vi "Filter Rendering.vi"() -> ()   [LabVIEW 2023]
doc: "Demonstrates how to use the DFD Render Transfer Function Equation VI, DFD Render Zero-Pole-Gain Equation VI, and DFD Render Difference Equation VI to present the characteristics of a filter in different graphs.\n\nComplete the following steps to use this VI.\n1) Run the VI.\n2) On the <B>Transfer Function Rendering</B> page, modify the <B>Transfer Function Display Format</B> option, and view the resulting transfer function. You also can modify the filter specifications.\n3) Click the <B>Zero-Pole-Gain Rendering</B> tab, modify the <B>Zero-Pole-Gain Equation Display Format</B> option, and view the resulting zero-pole-gain equation.\n4) Click the <B>Difference Equation Rendering</B> tab, modify the <B>Difference Equation Display Format</B> option, and view the resulting difference equation.\n5) Click the <B>STOP</B> button to stop this VI."
uses:
  <vilib>/addons/Digital Filter Design/_Objects.llb/DFD Filter Ripple Specification (Design).ctl
  <vilib>/addons/Digital Filter Design/_Objects.llb/DFD Filter Frequence Specification (Design).ctl
  <vilib>/addons/Digital Filter Design/NI_DigFilterLicensed.lvlib
panel:
  in  "Tab Control":T1(tab)
  out "Transfer Function":picture
  in  "Transfer Functions Display Format":u16(ring) items=["Expanded Form", " Second-Order Sections"]
  out "Zero-Pole-Gain Equation":picture
  in  "Zero-Pole-Gain Equation Display Format":u16(ring) items=["Separated Roots", "Combined Roots"]
  out "Difference Equation":picture
  in  "Difference Equation Display Format":u16(ring) items=["Feedback on left and feedforward on right", "Feedback and feedforward on right", "Feedback and feedforward on right in one line"]
  in  "Design Method":T2(ring)=enum."Elliptic"
  in  "Filter Type":u16(ring) items=["Lowpass", "Highpass", "Bandpass", "Bandstop"]
  in  "Frequency Sepcifications [Hz]":T3={"fpass 1"=250.0, "fstop 1"=400.0, "fpass 2 "=0.0, "fstop 2"=0.0}
  in  "Ripple Specifications":T4={"passband"=0.1, "stopband"=60.0, "dB/linear? (T: dB)"=TRUE}
  in  "Sampling Frequency [Hz]":dbl=1000.0 format="%.2f"
  in  "stop":bool
  out "Error Message":string
  # "Select Help>>Show Context Help and move the cursor over the VI icon for more information."
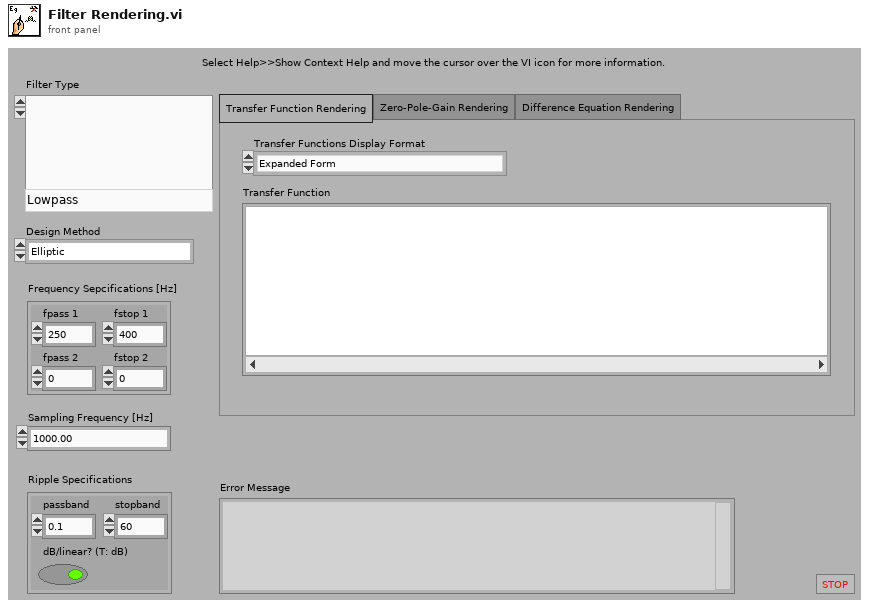
[diagram p1: front panel]
types:
  T1 = enum32{"Transfer Function Rendering", "Zero-Pole-Gain Rendering", "Difference Equation Rendering"}
  T2 = enum16{"Butterworth", "Chebyshev", "Inverse Chebyshev", "Elliptic", "Kaiser Window", "Dolph-Chebyshev Window", "Equi-Ripple FIR"}
  T3 = typedef "NI_DigFilterLicensed.lvlib/DFD Filter Frequence Specification (Design).ctl" = cluster{"fpass 1":dbl, "fstop 1":dbl, "fpass 2 ":dbl, "fstop 2":dbl}
  T4 = typedef "NI_DigFilterLicensed.lvlib/DFD Filter Ripple Specification (Design).ctl" = cluster{"passband":dbl, "stopband":dbl, "dB/linear? (T: dB)":bool}
  T5 = typedef "NI_DigFilterLicensed.lvlib/DFD Filter Obj.ctl" = cluster{"mSRate_Fs":dbl, "mSRate_Version":string, "mSRate_Comments":string, "mSRate_OrgCoef":T6, "mSRate_CurCoef":T6, "mSRate_Quantized?":bool, "mSRate_QCoef":T6, "mSRate_QSettings":T8[], "mSRate_Order":i32, "mSRate_Scaling":cluster{"mSRate_ScaleByPowerOf2?":bool, "mSRate_ScaleType":T10}}
  T6 = typedef "NI_DigFilterLicensed.lvlib/DFD Filter Coef.ctl" = cluster{"type":T7, "gain":dbl, "coef a (k)":dbl[], "coef b (v)":dbl[]}
  T7 = typedef "NI_DigFilterLicensed.lvlib/DFD Filter Structure Type Selector.ctl" = enum16{"Undefined", "FIR Direct Form", "FIR Direct Form Transposed", "FIR Symmetric", "FIR Antisymmetric", "IIR Direct Form I", "IIR Direct Form I Transposed", "IIR Direct Form II", "IIR Direct Form II Transposed", "IIR Cascaded Second Order Sections Form I", "IIR Cascaded Second Order Sections Form I Transposed", "IIR Cascaded Second Order Sections Form II", "IIR Cascaded Second Order Sections Form II Transposed", "Lattice Allpass (basic sections)", "Lattice Allpass (one multiplier sections)", "Lattice Allpass (normalized sections)", "Lattice AR (basic sections)", "Lattice AR (one multiplier sections)", "Lattice AR (normalized sections)", "Lattice MA (minimum phase)", "Lattice MA (maximum phase)", "Lattice ARMA (basic sections)", "Lattice ARMA (one multiplier sections)", "Lattice ARMA (normalized sections)"}
  T8 = typedef "NI_DigFilterLicensed.lvlib/dfd_Internal Quantization Settings.ctl" = cluster{"source":T9, "wl":i16, "iwl":i16, "overflow mode":enum16{"Saturation", "Wrap"}, "rounding mode":enum16{"Nearest", "Truncation"}, "signed?":bool}
  T9 = typedef "NI_DigFilterLicensed.lvlib/dfd_Internal Quantization Srcs.ctl" = u16
  T10 = typedef "NI_DigFilterLicensed.lvlib/DFD Coef Norm Type.ctl" = enum16{"No Norm", "Time Domain 1-Norm", "Time Domain 2-Norm", "Time Domain Inf-Norm"}
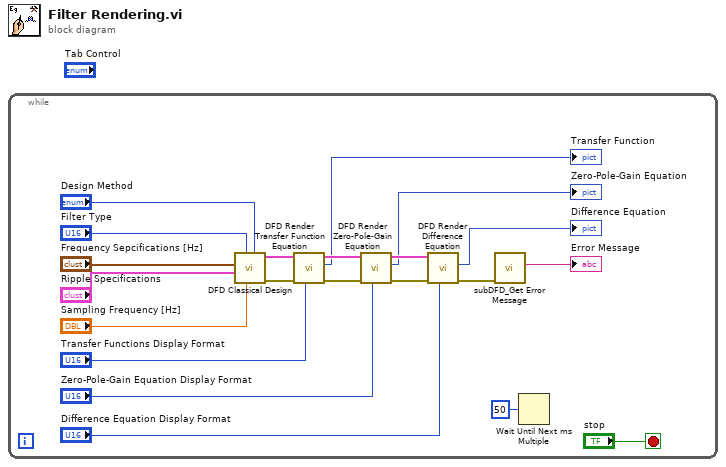
[diagram p0: block diagram]
diagram:
  n1 = while {
    stop <- "stop" stop-if-true
    n2 = call <vilib>:"DFD Classical Design.vi"("design method"="Design Method", "fs [Hz]"="Sampling Frequency [Hz]", "filter type"="Filter Type", "ripple specs"="Ripple Specifications", "freq specs [Hz]"="Frequency Sepcifications [Hz]") -> ("error out"=w3:errorcluster, "filter out"=w16:T5)  [unwired: 1 in, 4 out]
    n3 = call <vilib>:"DFD Render Transfer Function Equation.vi"("display format"="Transfer Functions Display Format", "error in (no error)"=w3, "filter in"=w16) -> ("error out"=w2:errorcluster, "transfer function"=→"Transfer Function":picture, "filter out"=w12:T5)  [unwired: 3 in, 3 out]
    n4 = call <vilib>:"DFD Render Zero-Pole-Gain Equation.vi"("display format"="Zero-Pole-Gain Equation Display Format", "error in (no error)"=w2, "filter in"=w12) -> ("error out"=w1:errorcluster, "zero-pole-gain equation"=→"Zero-Pole-Gain Equation":picture, "filter out"=w11:T5)  [unwired: 3 in, 3 out]
    n5 = call <vilib>:"DFD Render Difference Equation.vi"("display format"="Difference Equation Display Format", "error in (no error)"=w1, "filter in"=w11) -> ("error out"=w10:errorcluster, "difference equation"=→"Difference Equation":picture)  [unwired: 3 in, 4 out]
    n6 = call <vilib>:"subDFD_Get Error Message.vi"("error in (no error)"=w10) -> ("Error Message"=→"Error Message":string)  [unwired: 1 in, 9 out]
    n7 = Wait Until Next ms Multiple(millisecond multiple=u32 50) -> ()  [unwired: 1 out]
  }
